vi "CSM - Forward UI Operations to CSM.vi"(7 "Name (\"\" to Use UUID)":string, 9 "Error in":errorcluster caption="Error in (no error)", 10 "High Priority(T)":bool=TRUE, 11 "State(s) In (\"\")":string) -> (1 "Error out":errorcluster, 3 "States Out":string)   [LabVIEW 2017, in "Communicable State Machine.lvlib"]
doc: "Forwards events generated by user operations in a UI loop parallel to the CSM loop to the CSM loop for processing. This VI is primarily applied in Multi-Loop Mode. The CSM DQMH-Style Template VI also uses this logic.\n\n<b>Reference Example</b>: `Addons - Loop Support\\CSMLS - Continuous Loop in CSM Example.vi`.\n\n\n> [!NOTE] <b>CSM Multi-Loop Mode</b>\n>\n> In some scenarios, it is suitable to use multiple loops to constitute the same CSM module. For example:\n> - Retrofitting existing functional code into a CSM module. For example, TCP connection loops or DAQmx data acquisition loops. To ensure the clarity of the original logic, you can wrap the existing code in a While loop and append a CSM communication loop to implement the retrofitted functionality.\n> - In cases with high real-time requirements where a Timed Loop is needed, the CSM loop is required as a communication interface, while the Timed Loop serves as the functional loop implementation scheme.\n> - In cases where UI operations are very complex, it is recommended to separate UI operations from the CSM communication loop. The UI operation loop handles UI actions and generates inter-module messages, while the CSM loop serves as the actual functional loop.\n>\n> The Multi-Loop Support Mode API is used in such scenarios to pass internal messages between internal loops of a module or to provide CSM interface functionality for non-CSM loops.\n\n\n-- <b>Controls</b> --\n- <b>State(s) In (\"\")</b>: States to be processed.\n- <b>Name (\"\" to Use UUID)</b>: Module name.\n- <b>High Priority? (T)</b>: Immediate execution option. Sending immediately causes this message to be processed instantly in the CSM loop, rather than waiting for existing messages in the CSM loop to finish execution.\n\n-- <b>Indicators</b> --\n- <b>States Out</b>: Input is always empty. This output is set to ensure wire consistency in the template."
uses:
  Communicable State Machine.lvlib
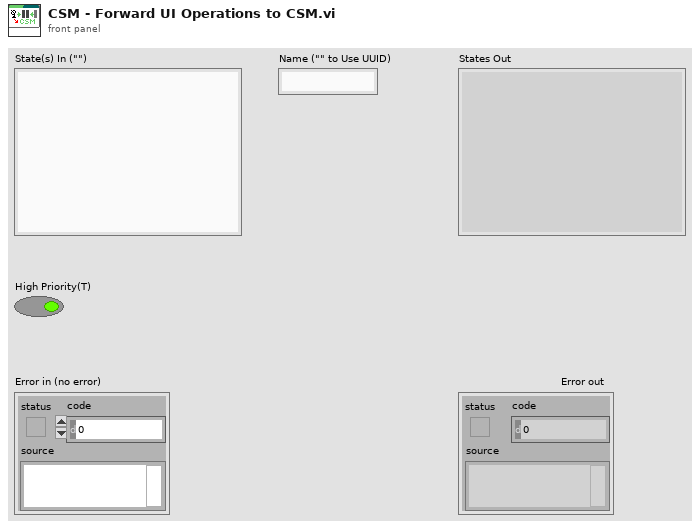
[diagram p1: front panel]
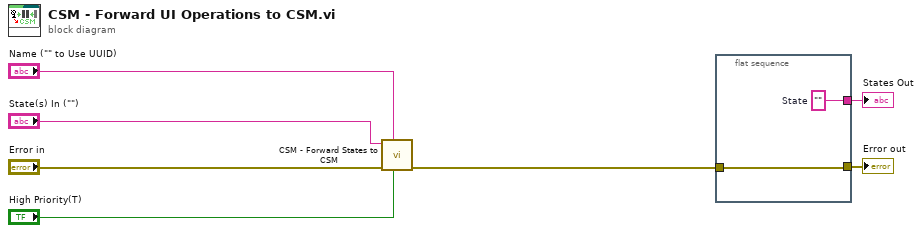
[diagram p0: block diagram]
diagram:
  n1 = call "CSM - Forward States to CSM.vi"("High Priority? (T)"="High Priority(T)", "Module Name"="Name (\"\" to Use UUID)", "Error In (No Error)"="Error in", "State (S) In (\"\")"="State(s) In (\"\")") -> ("error out"=w3:errorcluster)  [unwired: 7 in]
  n2 = flat-sequence {
    tunnel: [w9] -> w7
    tunnel: w3 -> [w8]
    tunnel: [w8] -> w1
    frame #0 {
      w9 = ""  # State
    }
  }
  "States Out" <- w7
  "Error out" <- w1
